vi "运维调试_五参数.vi"() -> ()   [LabVIEW 2016, in "斯坦道多参数.lvlib"]
uses:
  <vilib>/Utility/miscctls.llb/LVPointTypeDef.ctl
  <vilib>/Utility/config.llb/NI_LVConfig.lvlib
panel:
  in  "周期设置":bool
  in  "序号":string
  out "字符串":string
  out "运行状态":u16(ring) items=["空闲", "水样测试", "标样核查"]
  in  "叶绿素a校准":bool
  in  "停止":bool
  in  "标样核查":bool
  in  "水样测试":bool
  in  "open MB":bool
  in  "设置":bool
  in  "水温校准":bool
  in  "浊度校准":bool
  in  "溶解氧校准":bool
  in  "电导率校准":bool
  in  "pH校准":bool
  in  "探头校正返回":bool
  in  "探头校正":bool
  out "检测值":T1
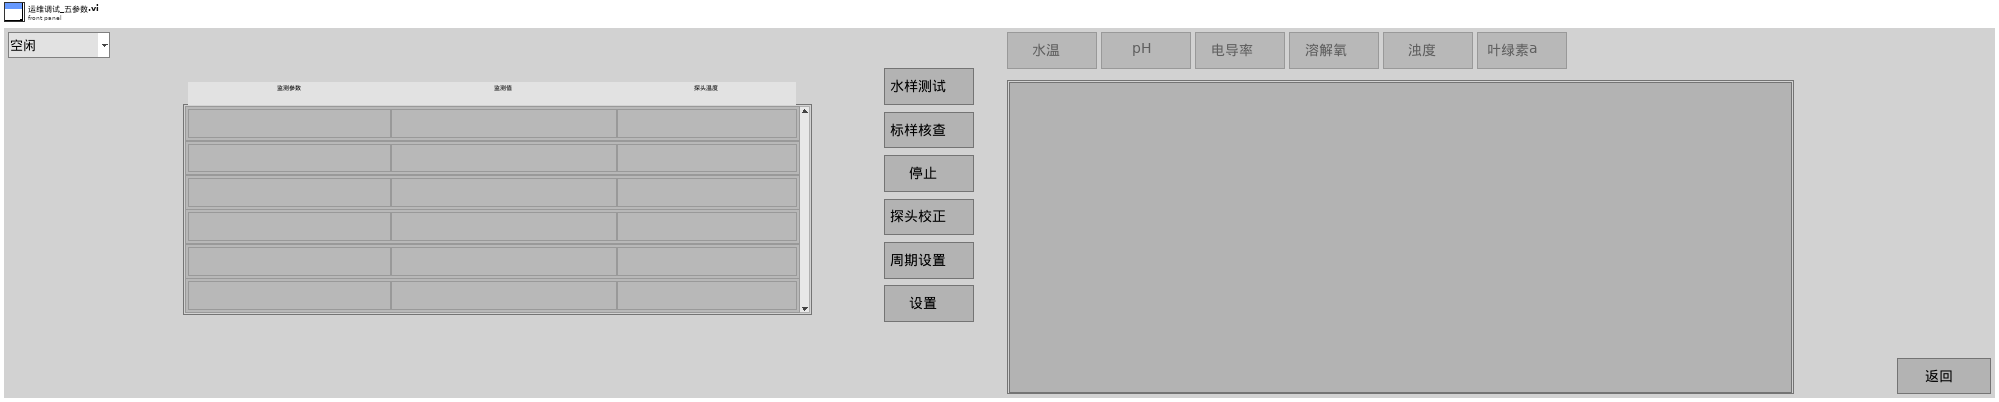
[diagram p1: front panel]
types:
  T1 = typedef "斯坦道多参数.lvlib/检测值.ctl" = cluster{"监测参数1":string, "浓度1":string, "探头温度1":string}[]
  T2 = typedef "LVPointTypeDef.ctl" = cluster{"Horizontal":i16, "Vertical":i16}
  T3 = cluster{"电极状态标志":u16, "电极型号标志":u16, "溶解氧测量值":sgl, "温度测量值":sgl, "溶解氧饱和度值":sgl, "盐度补偿值":sgl, "大气压补偿值":sgl, "溶解氧偏移修正值":sgl, "温度偏移修正值":sgl, "手动温度补偿值":sgl, "溶解氧电极零点":sgl, "溶解氧电极斜率":sgl, "第1点标准值记录":sgl, "第1点信号值记录":sgl, "第1点温度值记录":sgl, "第2点标准值记录":sgl, "第2点信号值记录":sgl, "第2点温度值记录":sgl, "命令滤波设定":u16, "温度模式":enum16{"ATC", "MTC"}, "生产批次":u16, "电极序号":u16, "串口地址":u16, "串口波特率":enum16{"9600", "19200", "115200"}, "串口校验位":enum16{"NONE", "ODD", "EVEN"}, "串口停止位":enum16{"1bit", "2bit"}, "第一点标准值":sgl, "第二点标准值":sgl}
  T4 = cluster{"电极状态标志":u16, "电极型号标志":u16, "酸碱度测量值":sgl, "温度测量值":sgl, "酸碱度信号值":sgl, "温度信号值":sgl, "酸碱度偏移修正值":sgl, "温度偏移修正值":sgl, "手动温度补偿值":sgl, "酸碱度电极零点":sgl, "酸碱度电极斜率":sgl, "第1点标准值记录":sgl, "第1点信号值记录":sgl, "第1点温度值记录":sgl, "第2点标准值记录":sgl, "第2点信号值记录":sgl, "第2点温度值记录":sgl, "命令滤波设定":u16, "温度模式":enum16{"ATC", "MTC"}, "生产批次":u16, "电极序号":u16, "串口地址":u16, "串口波特率":enum16{"9600", "19200", "115200"}, "串口校验位":enum16{"NONE", "ODD", "EVEN"}, "串口停止位":enum16{"1bit", "2bit"}, "第一点标准值":sgl, "第二点标准值":sgl}
  T5 = cluster{"电极状态标志":u16, "电极型号标志":u16, "浊度测量值":sgl, "温度测量值":sgl, "浊度信号值":sgl, "浊度偏移修正值":sgl, "温度偏移修正值":sgl, "手动温度补偿值":sgl, "浊度电极零点":sgl, "浊度电极斜率":sgl, "第1点标准值记录":sgl, "第1点信号值记录":sgl, "第1点温度值记录":sgl, "第2点标准值记录":sgl, "第2点信号值记录":sgl, "第2点温度值记录":sgl, "命令滤波设定":u16, "温度模式":enum16{"ATC", "MTC"}, "生产批次":u16, "电极序号":u16, "串口地址":u16, "串口波特率":enum16{"9600", "19200", "115200"}, "串口校验位":enum16{"NONE", "ODD", "EVEN"}, "串口停止位":enum16{"1bit", "2bit"}, "第一点标准值":sgl, "第二点标准值":sgl}
  T6 = cluster{"电极状态标志":u16, "电极型号标志":u16, "电导率测量值":sgl, "温度测量值":sgl, "电导率信号值":sgl, "温度信号值":sgl, "温度补偿系数":sgl, "电导率偏移修正值":sgl, "温度偏移修正值":sgl, "手动温度补偿值":sgl, "电导率电极零点":sgl, "电导率电极斜率":sgl, "命令滤波设定":u16, "温度模式":enum16{"ATC", "MTC"}, "生产批次":u16, "电极序号":u16, "串口地址":u16, "串口波特率":enum16{"9600", "19200", "115200"}, "串口校验位":enum16{"NONE", "ODD", "EVEN"}, "串口停止位":enum16{"1bit", "2bit"}, "第一点标准值":sgl, "第二点标准值":sgl}
  T7 = cluster{"监测参数1":string, "浓度1":string, "探头温度1":string}[]
  T8 = enum8{"Enabled", "Disabled", "Disabled and Grayed Out"}
  T9 = cluster{"CH":u16, "监测值":dbl, "监测信号值":dbl, "温度偏移修正值":sgl}
  T10 = typedef "NI_LVConfig.lvlib/Config Data RefNum.ctl" = refnum<k1>
  T11 = enum32{"Bad", "Idle", "Run top level", "Running"}
  T12 = enum32{"Invalid", "Standard", "Closed", "Hidden", "Minimized", "Maximized"}
  T13 = cluster{"数据保存间隔":dbl, "水温标样值":dbl, "pH标样值":dbl, "溶解氧标样值":dbl, "电导率标样值":dbl, "浊度标样值":dbl}
  T14 = cluster{"Temp":bool, "pH":bool, "DO":bool, "Cond":bool, "Turb":bool, "叶绿素a启用":bool, "蓝绿藻":bool}
  T15 = cluster{"baud rate (bps)":u32, "stop bits":u16, "parity":u16, "flow control":u16, "timeout":u32, "retries":i32}
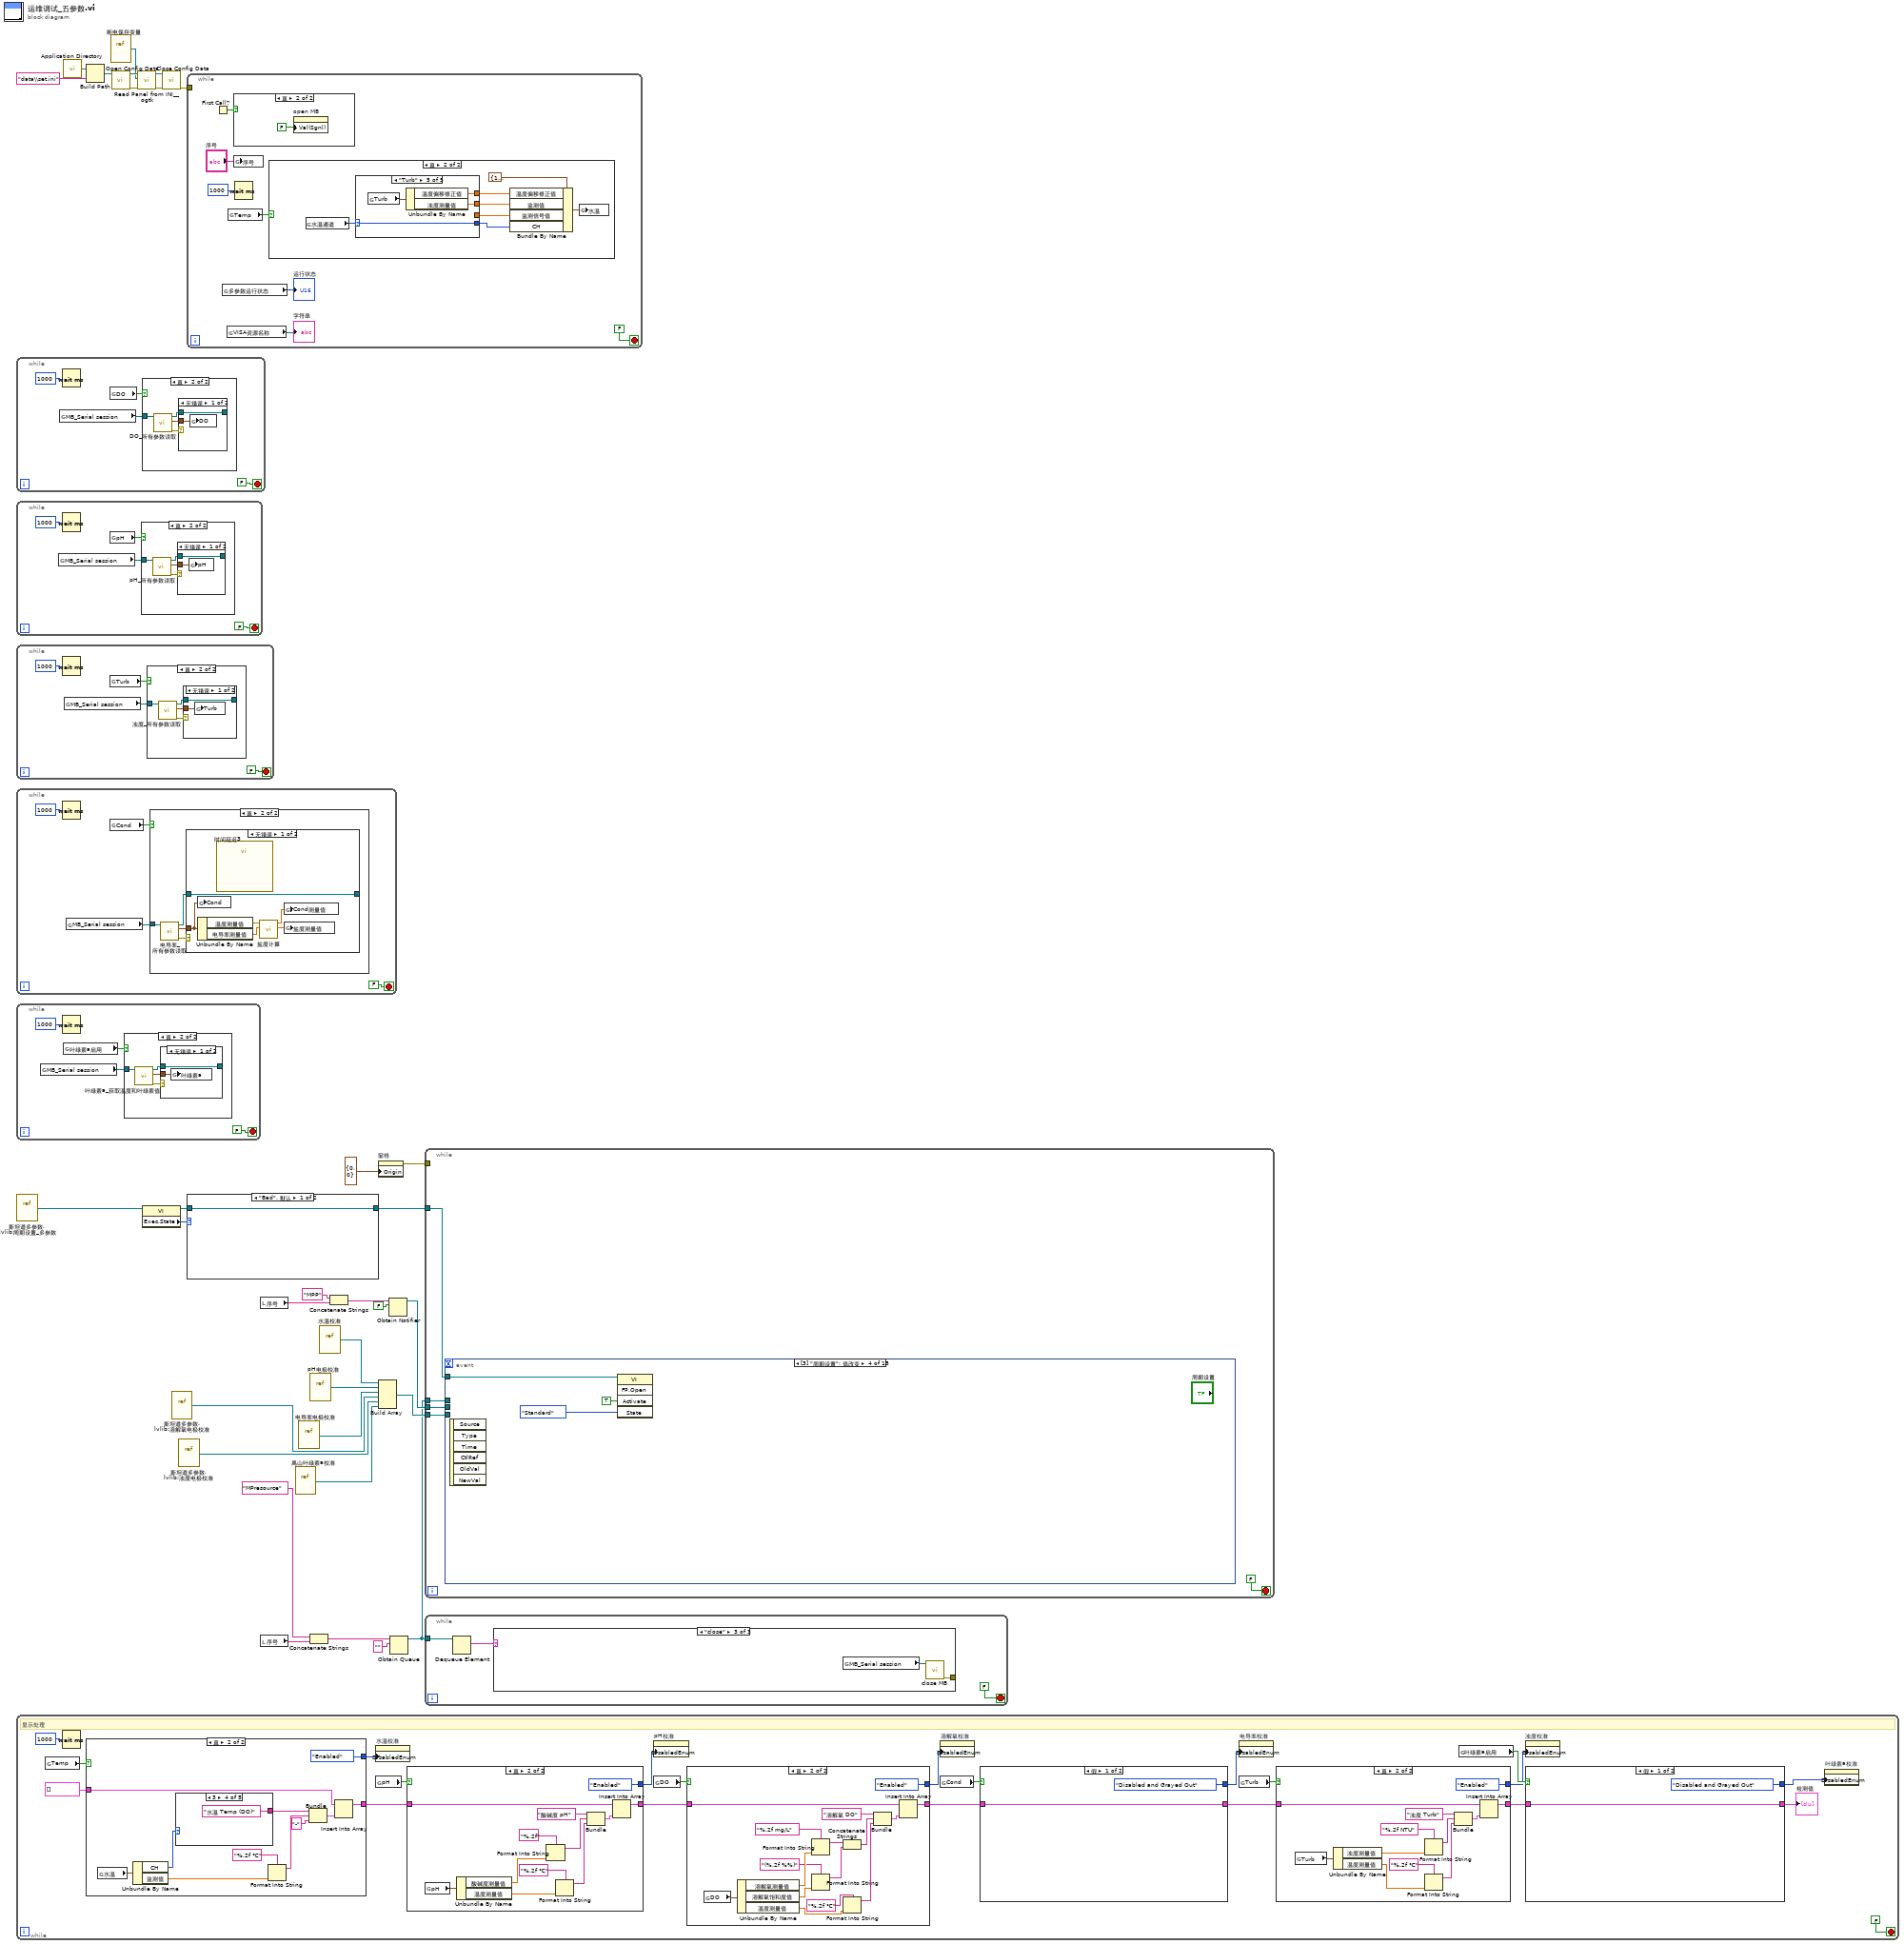
[diagram p0: block diagram]
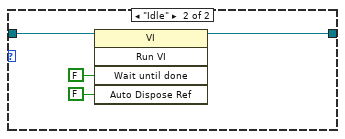
[diagram p2: hidden frame]
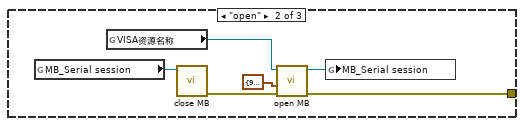
[diagram p4: hidden frame]
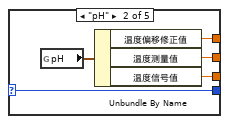
[diagram p17: hidden frame]
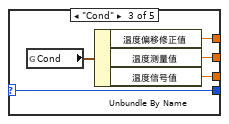
[diagram p18: hidden frame]
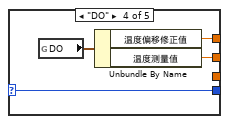
[diagram p19: hidden frame]
diagram:
  n1 = while {
    stop <- FALSE stop-if-true
    n2 = global read "多参数全局变量.vi" "MB_Serial session"() -> (w33:refnum<class "MB_Master_Serial.lvclass">)
    n3 = Wait (ms)(milliseconds to wait=u32 1000 ("等待时间（毫秒）")) -> ()  [unwired: 1 out]
    n4 = global read "断电保存变量.vi" "DO"() -> (w34:bool)
    n5 = case shown="真" w34 {
      tunnel: w33 -> [_ w37]
      frame False {
      }
      frame True {
        n6 = call "DO_所有参数读取.vi"("MB_Serial session in"=w37) -> ("error out"=w39:errorcluster, "输出值"=w40:T3, "MB_Serial session out"=w38:refnum<class "MB_Master_Serial.lvclass">)  [unwired: 8 in]
        n7 = case shown="无错误" w39 {
          tunnel: w40 -> [w41 _]
          tunnel: w38 -> [w42 w43]
          tunnel: [w42 w43] -> _
          frame No Error {
            n8 = global write "国弘过程全局变量.vi" "DO"(w41) -> ()
          }
          frame Error {
          }
        }
      }
    }
  }
  n9 = while {
    stop <- FALSE stop-if-true
    n10 = global read "多参数全局变量.vi" "MB_Serial session"() -> (w44:refnum<class "MB_Master_Serial.lvclass">)
    n11 = Wait (ms)(milliseconds to wait=u32 1000 ("等待时间（毫秒）")) -> ()  [unwired: 1 out]
    n12 = global read "断电保存变量.vi" "pH"() -> (w46:bool)
    n13 = case shown="真" w46 {
      tunnel: w44 -> [_ w48]
      frame False {
      }
      frame True {
        n14 = call "pH_所有参数读取.vi"("MB_Serial session in"=w48) -> ("error out"=w50:errorcluster, "输出值"=w51:T4, "MB_Serial session out"=w49:refnum<class "MB_Master_Serial.lvclass">)  [unwired: 8 in]
        n15 = case shown="无错误" w50 {
          tunnel: w51 -> [w53 _]
          tunnel: w49 -> [w52 w54]
          tunnel: [w52 w54] -> _
          frame No Error {
            n16 = global write "国弘过程全局变量.vi" "pH"(w53) -> ()
          }
          frame Error {
          }
        }
      }
    }
  }
  n17 = while {
    stop <- FALSE stop-if-true
    n18 = Wait (ms)(milliseconds to wait=u32 1000 ("等待时间（毫秒）")) -> ()  [unwired: 1 out]
    n19 = global read "多参数全局变量.vi" "MB_Serial session"() -> (w55:refnum<class "MB_Master_Serial.lvclass">)
    n20 = global read "断电保存变量.vi" "Turb"() -> (w57:bool)
    n21 = case shown="真" w57 {
      tunnel: w55 -> [_ w59]
      frame False {
      }
      frame True {
        n22 = call "浊度_所有参数读取.vi"("MB_Serial session in"=w59) -> ("error out"=w61:errorcluster, "输出值"=w62:T5, "MB_Serial session out"=w60:refnum<class "MB_Master_Serial.lvclass">)  [unwired: 8 in]
        n23 = case shown="无错误" w61 {
          tunnel: w62 -> [w63 _]
          tunnel: w60 -> [w64 w65]
          tunnel: [w64 w65] -> _
          frame No Error {
            n24 = global write "国弘过程全局变量.vi" "Turb"(w63) -> ()
          }
          frame Error {
          }
        }
      }
    }
  }
  n25 = while {
    stop <- FALSE stop-if-true
    n26 = Wait (ms)(milliseconds to wait=u32 1000 ("等待时间（毫秒）")) -> ()  [unwired: 1 out]
    n27 = global read "多参数全局变量.vi" "MB_Serial session"() -> (w66:refnum<class "MB_Master_Serial.lvclass">)
    n28 = global read "断电保存变量.vi" "Cond"() -> (w68:bool)
    n29 = case shown="真" w68 {
      tunnel: w66 -> [_ w70]
      frame False {
      }
      frame True {
        n30 = call "电导率_所有参数读取.vi"("MB_Serial session in"=w70) -> ("error out"=w72:errorcluster, "输出值"=w73:T6, "MB_Serial session out"=w71:refnum<class "MB_Master_Serial.lvclass">)  [unwired: 8 in]
        n31 = case shown="无错误" w72 {
          tunnel: w73 -> [w78 _]
          tunnel: [w79 w80] -> _
          tunnel: w71 -> [w79 w80]
          frame No Error {
            n32 = global write "国弘过程全局变量.vi" "Cond"(w78) -> ()
            n33 = Unbundle By Name(w78) -> ("温度测量值"=w76:sgl, "电导率测量值"=w77:sgl)
            n34 = call "时间延迟3"() -> ()  [unwired: 11 in, 1 out]
            n35 = call "盐度计算.vi"("spCond"=w77, "Temp"=w76) -> ("saltresult"=w74:dbl, "cond"=w75:dbl)  [unwired: 8 in]
            n36 = global write "国弘过程全局变量.vi" "Cond测量值"(w75) -> ()
            n37 = global write "国弘过程全局变量.vi" "盐度测量值"(w74) -> ()
          }
          frame Error {
          }
        }
      }
    }
  }
  n38 = while {
    stop <- FALSE stop-if-true
    n39 = global read "多参数全局变量.vi" "MB_Serial session"() -> (w81:refnum<class "MB_Master_Serial.lvclass">)
    n40 = Wait (ms)(milliseconds to wait=u32 1000 ("等待时间（毫秒）")) -> ()  [unwired: 1 out]
    n41 = global read "断电保存变量.vi" "叶绿素a启用"() -> (w83:bool)
    n42 = case shown="真" w83 {
      tunnel: w81 -> [_ w85]
      frame False {
      }
      frame True {
        n43 = call "叶绿素a_获取温度和叶绿素值.vi"("MB_Serial session in"=w85) -> ("error out"=w87:errorcluster, "输出值"=w88:cluster{"温度测量值":sgl, "叶绿素测量值":sgl, "错误标志":u16}, "MB_Serial session out"=w86:refnum<class "MB_Master_Serial.lvclass">)  [unwired: 8 in]
        n44 = case shown="无错误" w87 {
          tunnel: w88 -> [w89 _]
          tunnel: w86 -> [w90 w91]
          tunnel: [w90 w91] -> _
          frame No Error {
            n45 = global write "禹山过程全局变量.vi" "叶绿素a"(w89) -> ()
          }
          frame Error {
          }
        }
      }
    }
  }
  n46 = vi-ref "斯坦道多参数.lvlib:周期设置_多参数.vi"() -> (w4:refnum<vi>)
  n47 = while {
    stop <- FALSE stop-if-true
    # "显示处理"
    n48 = global read "断电保存变量.vi" "Temp"() -> (w110:bool)
    n49 = Wait (ms)(milliseconds to wait=u32 1000 ("等待时间（毫秒）")) -> ()  [unwired: 1 out]
    n50 = case shown="真" w110 {
      tunnel: [w188 w190] -> w107
      tunnel: T7 [] ("数组") -> [w188 w191]
      tunnel: [T8."Disabled and Grayed Out" ("禁用") T8."Enabled" ("禁用")] -> w92
      frame False {
      }
      frame True {
        n51 = global read "国弘过程全局变量.vi" "水温"() -> (w199:T9)
        n52 = Unbundle By Name(w199) -> ("CH"=w196:u16, "监测值"=w197:dbl)
        n53 = case shown="3" w196 {
          tunnel: ["水温 Temp" ("监测参数1") "水温 Temp (pH)" ("监测参数1") "水温 Temp (Cond)" ("监测参数1") "水温 Temp (DO)" ("监测参数1") "水温 Temp (Turb)" ("监测参数1")] -> w195
          frame 0, Default {
          }
          frame 1 {
          }
          frame 2 {
          }
          frame 3 {
          }
          frame 4 {
          }
        }
        n54 = Format Into String(format string="%.2f ℃" ("格式字符串"), w197) -> (resulting string=w194:string)  [unwired: 2 in, 1 out]
        n55 = Bundle("监测参数1"=w195, w194, "探头温度1"="-") -> (w192:cluster{"监测参数1":string, string, "探头温度1":string})  [unwired: 1 in]
        n56 = Insert Into Array(array=w191, new element=w192) -> (w190:T7)  [unwired: 1 in]
      }
    }
    n57 = property on="水温校准" class="Bool"("DisabledEnum"=w92) -> ()  [unwired: 2 in, 2 out]
    n58 = global read "断电保存变量.vi" "pH"() -> (w108:bool)
    n59 = case shown="真" w108 {
      tunnel: [w174 w176] -> w105
      tunnel: w107 -> [w174 w178]
      tunnel: [T8."Disabled and Grayed Out" ("禁用") T8."Enabled" ("禁用")] -> w97
      frame False {
      }
      frame True {
        n60 = global read "国弘过程全局变量.vi" "pH"() -> (w186:T4)
        n61 = Unbundle By Name(w186) -> ("酸碱度测量值"=w185:sgl, "温度测量值"=w183:sgl)
        n62 = Format Into String(format string="%.2f" ("格式字符串"), w185) -> (resulting string=w179:string)  [unwired: 2 in, 1 out]
        n63 = Format Into String(format string="%.2f ℃" ("格式字符串"), w183) -> (resulting string=w181:string)  [unwired: 2 in, 1 out]
        n64 = Bundle("监测参数2"="酸碱度 pH", w179, w181) -> (w177:cluster{"监测参数2":string, string, string})  [unwired: 1 in]
        n65 = Insert Into Array(array=w178, new element=w177) -> (w176:T7)  [unwired: 1 in]
      }
    }
    n66 = property on="pH校准" class="Bool"("DisabledEnum"=w97) -> ()  [unwired: 2 in, 2 out]
    n67 = global read "断电保存变量.vi" "DO"() -> (w106:bool)
    n68 = case shown="真" w106 {
      tunnel: [w156 w159] -> w102
      tunnel: w105 -> [w156 w160]
      tunnel: [T8."Disabled and Grayed Out" ("禁用") T8."Enabled" ("禁用")] -> w96
      frame False {
      }
      frame True {
        n69 = global read "国弘过程全局变量.vi" "DO"() -> (w157:T3)
        n70 = Unbundle By Name(w157) -> ("溶解氧测量值"=w169:sgl, "溶解氧饱和度值"=w167:sgl, "温度测量值"=w171:sgl)
        n71 = Format Into String(format string="%.2f mg/L" ("格式字符串"), w169) -> (resulting string=w166:string)  [unwired: 2 in, 1 out]
        n72 = Format Into String(format string="(%.2f %%)" ("格式字符串"), w167) -> (resulting string=w165:string)  [unwired: 2 in, 1 out]
        n73 = Concatenate Strings(w166, w165) -> (w164:string)
        n74 = Format Into String(format string="%.2f ℃" ("格式字符串"), w171) -> (resulting string=w162:string)  [unwired: 2 in, 1 out]
        n75 = Bundle("监测参数2"="溶解氧 DO", w164, w162) -> (w161:cluster{"监测参数2":string, string, string})  [unwired: 1 in]
        n76 = Insert Into Array(array=w160, new element=w161) -> (w159:T7)  [unwired: 1 in]
      }
    }
    n77 = property on="溶解氧校准" class="Bool"("DisabledEnum"=w96) -> ()  [unwired: 2 in, 2 out]
    n78 = global read "断电保存变量.vi" "Cond"() -> (w104:bool)
    n79 = case shown="假" w104 {
      tunnel: w102 -> [w142 w146]
      tunnel: [w142 w144] -> w101
      tunnel: [T8."Disabled and Grayed Out" ("禁用") T8."Enabled" ("禁用")] -> w95
      frame False {
      }
      frame True {
        n80 = global read "国弘过程全局变量.vi" "Cond"() -> (w154:T6)
        n81 = Unbundle By Name(w154) -> ("电导率测量值"=w153:sgl, "温度测量值"=w151:sgl)
        n82 = Format Into String(format string="%.2f uS/cm" ("格式字符串"), w153) -> (resulting string=w147:string)  [unwired: 2 in, 1 out]
        n83 = Format Into String(format string="%.2f ℃" ("格式字符串"), w151) -> (resulting string=w148:string)  [unwired: 2 in, 1 out]
        n84 = Bundle("监测参数2"="电导率 Cond", w147, w148) -> (w145:cluster{"监测参数2":string, string, string})  [unwired: 1 in]
        n85 = Insert Into Array(array=w146, new element=w145) -> (w144:T7)  [unwired: 1 in]
      }
    }
    n86 = property on="电导率校准" class="Bool"("DisabledEnum"=w95) -> ()  [unwired: 2 in, 2 out]
    n87 = global read "断电保存变量.vi" "Turb"() -> (w103:bool)
    n88 = case shown="真" w103 {
      tunnel: w101 -> [w128 w133]
      tunnel: [w128 w131] -> w100
      tunnel: [T8."Disabled and Grayed Out" ("禁用") T8."Enabled" ("禁用")] -> w94
      frame False {
      }
      frame True {
        n89 = global read "国弘过程全局变量.vi" "Turb"() -> (w129:T5)
        n90 = Unbundle By Name(w129) -> ("浊度测量值"=w137:sgl, "温度测量值"=w139:sgl)
        n91 = Format Into String(format string="%.2f NTU" ("格式字符串"), w137) -> (resulting string=w135:string)  [unwired: 2 in, 1 out]
        n92 = Format Into String(format string="%.2f ℃" ("格式字符串"), w139) -> (resulting string=w136:string)  [unwired: 2 in, 1 out]
        n93 = Bundle("监测参数2"="浊度 Turb", w135, w136) -> (w132:cluster{"监测参数2":string, string, string})  [unwired: 1 in]
        n94 = Insert Into Array(array=w133, new element=w132) -> (w131:T7)  [unwired: 1 in]
      }
    }
    n95 = global read "断电保存变量.vi" "叶绿素a启用"() -> (w98:bool)
    n96 = property on="浊度校准" class="Bool"("DisabledEnum"=w94) -> ()  [unwired: 2 in, 2 out]
    n97 = case shown="假" w98 {
      tunnel: w100 -> [w114 w121]
      tunnel: [w114 w119] -> w99
      tunnel: [T8."Disabled and Grayed Out" ("禁用") T8."Enabled" ("禁用")] -> w93
      frame False {
      }
      frame True {
        n98 = global read "禹山过程全局变量.vi" "叶绿素a"() -> (w118:cluster{"温度测量值":sgl, "叶绿素测量值":sgl, "错误标志":u16})
        n99 = Unbundle By Name(w118) -> ("叶绿素测量值"=w117:sgl, "温度测量值"=w116:sgl)
        n100 = Format Into String(format string="%.2f ug/L" ("格式字符串"), w117) -> (resulting string=w123:string)  [unwired: 2 in, 1 out]
        n101 = Format Into String(format string="%.2f ℃" ("格式字符串"), w116) -> (resulting string=w124:string)  [unwired: 2 in, 1 out]
        n102 = Bundle("监测参数2"="叶绿素a Chla", w123, w124) -> (w120:cluster{"监测参数2":string, string, string})  [unwired: 1 in]
        n103 = Insert Into Array(array=w121, new element=w120) -> (w119:T7)  [unwired: 1 in]
      }
    }
    "检测值" <- w99
    n104 = property on="叶绿素a校准" class="Bool"("DisabledEnum"=w93) -> ()  [unwired: 2 in, 2 out]
  }
  n105 = call <vilib>:"Application Directory.vi"() -> ("Application Directory"=w20:path)
  n106 = Build Path(base path=w20, name or relative path="data\\set.ini" ("名称或相对路径")) -> (appended path=w19:path)
  n107 = vi-ref "断电保存变量.vi"() -> (w17:refnum<vi>)
  n108 = call <vilib>:"Open Config Data.vi"("configuration file path"=w19) -> ("error out"=w23:errorcluster, "refnum"=w24:T10)  [unwired: 8 in, 1 out]
  n109 = call <userlib>:"Read Panel from INI__ogtk.vi"("error in (no error)"=w23, "VI ref"=w17, "refnum"=w24) -> ("error out"=w21:errorcluster, "refnum out"=w22:T10)  [unwired: 7 in]
  n110 = property class="VI"(reference=w4) -> (reference out=w2:refnum<vi>, "Exec.State"=w3:T11)  [unwired: 1 in, 1 out]
  n111 = call <vilib>:"Close Config Data.vi"("error in (no error)"=w21, "refnum"=w22) -> ("error out"=w16:errorcluster)  [unwired: 8 in, 1 out]
  n112 = vi-ref "斯坦道多参数.lvlib:溶解氧电极校准.vi"() -> (w26:refnum<vi>)
  n113 = vi-ref "斯坦道多参数.lvlib:浊度电极校准.vi"() -> (w25:refnum<vi>)
  n114 = while {
    tunnel: w16 -> [_]
    stop <- FALSE stop-if-true
    n115 = First Call?() -> (First Call?: T/F=w209:bool)
    n116 = global read "多参数全局变量.vi" "多参数运行状态"() -> (→"运行状态":u16)
    n117 = global read "断电保存变量.vi" "VISA资源名称"() -> (→"字符串":refnum<visa-resource-name>)
    n118 = global read "断电保存变量.vi" "Temp"() -> (w208:bool)
    n119 = case shown="真" w209 {
      frame False {
      }
      frame True {
        n120 = property on="open MB" class="Bool (严格)"("Val(Sgnl)"=FALSE ("值(信号)")) -> ()  [unwired: 2 in, 2 out]
      }
    }
    n121 = global write "多参数全局变量.vi" "序号"("序号") -> ()
    n122 = Wait (ms)(milliseconds to wait=u32 1000 ("等待时间（毫秒）")) -> ()  [unwired: 1 out]
    n123 = case shown="真" w208 {
      frame False {
      }
      frame True {
        n124 = global read "断电保存变量.vi" "水温通道"() -> (w218:enum16{"NULL", "pH", "Cond", "DO", "Turb"})
        n125 = case shown="\"Turb\"" w218 {
          selector: w218 -> [w219 w224 w229 w233 w237]
          tunnel: [w219 w224 w229 w233 w237] -> w217
          tunnel: [_ w222 w227 w230 w235] -> w216
          tunnel: [_ w221 w226 _ _] -> w215
          tunnel: [_ w220 w225 w231 w234] -> w212
          frame "NULL", Default {
          }
          frame "pH" {
            n126 = global read "国弘过程全局变量.vi" "pH"() -> (w223:T4)
            n127 = Unbundle By Name(w223) -> ("温度偏移修正值"=w220:sgl, "温度测量值"=w222:sgl, "温度信号值"=w221:sgl)
          }
          frame "Cond" {
            n128 = global read "国弘过程全局变量.vi" "Cond"() -> (w228:T6)
            n129 = Unbundle By Name(w228) -> ("温度偏移修正值"=w225:sgl, "温度测量值"=w227:sgl, "温度信号值"=w226:sgl)
          }
          frame "DO" {
            n130 = global read "国弘过程全局变量.vi" "DO"() -> (w232:T3)
            n131 = Unbundle By Name(w232) -> ("温度偏移修正值"=w231:sgl, "温度测量值"=w230:sgl)
          }
          frame "Turb" {
            n132 = global read "国弘过程全局变量.vi" "Turb"() -> (w236:T5)
            n133 = Unbundle By Name(w236) -> ("温度偏移修正值"=w234:sgl, "浊度测量值"=w235:sgl)
          }
        }
        n134 = Bundle By Name(cluster=T9 {"CH"=1, "监测值"=0.0, "监测信号值"=0.0, "温度偏移修正值"=0.0} ("水温"), "温度偏移修正值"=w212, "监测值"=w216, "监测信号值"=w215, "CH"=w217) -> (w214:T9)
        n135 = global write "国弘过程全局变量.vi" "水温"(w214) -> ()
      }
    }
  }
  n136 = case shown="\"Bad\", 默认" w3 {
    tunnel: w2 -> [w239 w243]
    tunnel: [w239 w240] -> w1
    frame "Bad", Default {
    }
    frame "Idle" {
      n137 = invoke class="VI" method="Run VI"(reference=w243, "Wait until done"=FALSE ("结束前等待"), "Auto Dispose Ref"=FALSE ("自动销毁引用")) -> (reference out=w240:refnum<vi>)  [unwired: 2 in, 4 out]
    }
  }
  n138 = local read "序号"() -> (w6:string)
  n139 = local read "序号"() -> (w5:string)
  n140 = vi-ref "禹山叶绿素a校准.vi"() -> (w15:refnum<vi>)
  n141 = vi-ref "电导率电极校准.vi"() -> (w27:refnum<vi>)
  n142 = Concatenate Strings("MPresource" ("名称（未命名）"), w5) -> (w7:string)
  n143 = vi-ref "pH电极校准.vi"() -> (w28:refnum<vi>)
  n144 = vi-ref "水温校准.vi"() -> (w29:refnum<vi>)
  n145 = Concatenate Strings("MPP" ("名称（未命名）"), w6) -> (w8:string)
  n146 = property on="窗格" class="Pane"("Origin"=T2 {"Horizontal"=0, "Vertical"=0} ("原点")) -> (error out=w32:errorcluster)  [unwired: 2 in, 1 out]
  n147 = Build Array(w29, w28, w27, w26, w25, w15) -> (w30:refnum<vi>[])
  n148 = Obtain Notifier(name (unnamed)=w8, notification data type=FALSE) -> (notifier out=w12:refnum<notifier>)  [unwired: 2 in, 2 out]
  n149 = Obtain Queue(name (unnamed)=w7, element data type="" ("名称（未命名）")) -> (queue out=w9:refnum<queue>)  [unwired: 3 in, 2 out]
  n150 = while {
    tunnel: w32 -> [_]
    tunnel: w30 -> [w247]
    tunnel: w12 -> [w246]
    tunnel: w9 -> [w245]
    tunnel: w1 -> [w244]
    stop <- FALSE stop-if-true
    n151 = event shown="[3] \"周期设置\": 值改变" {
      selector: _ -> [_ _ _ _ _ _ _ _ _ _ _ _ _ _ _]
      dyn-events: _ -> [_ _ _ _ _ _ _ _ _ _ _ _ _ _ _]
      timeout: _ -> [_ _ _ _ _ _ _ _ _ _ _ _ _ _ _]
      tunnel: w247 -> [_ _ _ _ _ _ _ w310 w323 w336 w348 w360 w372 w384 w396]
      tunnel: w246 -> [_ _ _ _ w283 _ _ _ _ _ _ _ _ _ _]
      tunnel: w245 -> [_ _ _ _ _ w286 _ _ _ _ _ _ _ _ _]
      tunnel: w244 -> [_ _ _ w281 _ _ _ _ _ _ _ _ _ _ _]
      event Timeout {
        n152 = event-data() -> ()  [unwired: 1 in, 3 out]
      }
      event "水样测试": Value Change {
        n153 = event-data() -> ()  [unwired: 1 in, 6 out]
        n154 = call "水样测试配置.vi"() -> ("确认输出"=w250:bool, "水样测定时间输出"=w249:dbl)  [unwired: 10 in]
        n155 = case shown="真" w250 {
          tunnel: w249 -> [_ w253]
          frame False {
          }
          frame True {
            n156 = vi-ref "水样测试.vi"() -> (w254:refnum<vi>)
            n157 = property class="VI"(reference=w254) -> ("Name"=w258:string, "Exec.State"=w256:T11)  [unwired: 1 in, 2 out]
            n158 = Open VI Reference(type specifier VI Refnum (for type only)=refnum<vi> refnum, vi path=w258, options=128 ("选项")) -> (vi reference=w259:refnum<vi>)  [unwired: 3 in, 1 out]
            n159 = case shown="\"Idle\"" w256 {
              tunnel: [w260 w264] -> w255
              tunnel: w259 -> [w260 w263]
              tunnel: w253 -> [_ w262]
              tunnel: "hd" ("数据标记表") -> [_ w261]
              frame "Bad", Default {
              }
              frame "Idle" {
                n160 = call-by-ref "开始异步调用"(reference=w263, "数据标记表"=w261, "水样测试时间"=w262) -> (reference out=w264:refnum<vi>)  [unwired: 11 in, 1 out]
              }
            }
            n161 = Close Reference(reference=w255) -> ()  [unwired: 1 in, 1 out]
          }
        }
      }
      event "标样核查": Value Change {
        n162 = event-data() -> ()  [unwired: 1 in, 6 out]
        n163 = call "标样核查配置.vi"() -> ("确认输出"=w266:bool, "标样核查配置"=w265:T13)  [unwired: 10 in]
        n164 = case shown="真" w266 {
          tunnel: w265 -> [_ w267]
          frame False {
          }
          frame True {
            n165 = vi-ref "标样核查.vi"() -> (w268:refnum<vi>)
            n166 = property class="VI"(reference=w268) -> ("Name"=w273:string, "Exec.State"=w270:T11)  [unwired: 1 in, 2 out]
            n167 = Open VI Reference(type specifier VI Refnum (for type only)=refnum<vi> refnum, vi path=w273, options=128 ("选项")) -> (vi reference=w274:refnum<vi>)  [unwired: 3 in, 1 out]
            n168 = case shown="\"Idle\"" w270 {
              tunnel: [w275 w278] -> w269
              tunnel: w274 -> [w275 w277]
              tunnel: w267 -> [_ w276]
              frame "Bad", Default {
              }
              frame "Idle" {
                n169 = call-by-ref "开始异步调用"(reference=w277, "标样核查配置"=w276) -> (reference out=w278:refnum<vi>)  [unwired: 12 in, 1 out]
              }
            }
            n170 = Close Reference(reference=w269) -> ()  [unwired: 1 in, 1 out]
          }
        }
      }
      event "周期设置": Value Change {
        n171 = event-data() -> ()  [unwired: 1 in, 6 out]
        n172 = invoke class="VI" method="FP.Open"(reference=w281, "Activate"=TRUE ("激活？"), "State"=T12."Standard" ("状态")) -> ()  [unwired: 2 in, 5 out]
      }
      event "停止": Value Change {
        n173 = event-data() -> ()  [unwired: 1 in, 6 out]
        n174 = Send Notification(notification=TRUE ("通知"), notifier=w283) -> ()  [unwired: 1 in, 2 out]
      }
      event "open MB": Value Change {
        n175 = event-data() -> ()  [unwired: 1 in, 6 out]
        n176 = Flush Queue(queue=w286) -> (queue out=w285:refnum<queue>)  [unwired: 1 in, 2 out]
        n177 = Enqueue Element(queue=w285, element="open" ("元素")) -> ()  [unwired: 2 in, 3 out]
      }
      event "设置": Value Change {
        n178 = event-data() -> ()  [unwired: 1 in, 6 out]
        n179 = flat-sequence {
          frame #0 {
            n180 = call "配置.vi"() -> ("启用参数"=w294:T14, "串口输出"=w295:refnum<visa-resource-name>)  [unwired: 10 in]
            n181 = global write "断电保存变量.vi" "VISA资源名称"(w295) -> ()
            n182 = Unbundle By Name(w294) -> ("Temp"=w289:bool, "pH"=w290:bool, "DO"=w291:bool, "Cond"=w292:bool, "Turb"=w293:bool, "叶绿素a启用"=w288:bool, "蓝绿藻"=w287:bool)
            n183 = global write "断电保存变量.vi" "pH"(w290) -> ()
            n184 = global write "断电保存变量.vi" "DO"(w291) -> ()
            n185 = global write "断电保存变量.vi" "Cond"(w292) -> ()
            n186 = global write "断电保存变量.vi" "Turb"(w293) -> ()
            n187 = global write "断电保存变量.vi" "Temp"(w289) -> ()
            n188 = global write "断电保存变量.vi" "叶绿素a启用"(w288) -> ()
            n189 = global write "断电保存变量.vi" "蓝绿藻"(w287) -> ()
          }
          frame #1 {
            n190 = call <vilib>:"Application Directory.vi"() -> ("Application Directory"=w305:path)
            n191 = Build Path(base path=w305, name or relative path="data\\set.ini" ("名称或相对路径")) -> (appended path=w304:path)
            n192 = call <vilib>:"Open Config Data.vi"("configuration file path"=w304) -> ("error out"=w308:errorcluster, "refnum"=w309:T10)  [unwired: 8 in, 1 out]
            n193 = vi-ref "断电保存变量.vi"() -> (w302:refnum<vi>)
            n194 = call <userlib>:"Write Panel to INI__ogtk.vi"("error in (no error)"=w308, "VI ref"=w302, "refnum"=w309) -> ("error out"=w306:errorcluster, "refnum out"=w307:T10)  [unwired: 7 in]
            n195 = call <vilib>:"Close Config Data.vi"("error in (no error)"=w306, "refnum"=w307) -> ("error out"=w298:errorcluster, "file path"=w299:path)  [unwired: 8 in]
            n196 = Open/Create/Replace File(file path (use dialog)=w299, error in=w298) -> (refnum out=w300:refnum<file>, error out=w301:errorcluster)  [unwired: 4 in, 1 out]
            n197 = Flush File(refnum=w300, error in=w301) -> (refnum out=w296:refnum<file>, error out=w297:errorcluster)
            n198 = Close File(refnum=w296, error in=w297) -> ()  [unwired: 2 out]
          }
          frame #2 {
          }
        }
      }
      event "探头校正返回": Value Change {
        n199 = event-data() -> ()  [unwired: 1 in, 6 out]
        n200 = property on="窗格" class="Pane"("Origin"=T2 {"Horizontal"=0, "Vertical"=0} ("原点")) -> ()  [unwired: 2 in, 2 out]
        n201 = disable-structure shown="禁用" {
          disable-tunnel: w310 -> [w312 _]
          frame Disabled {
            n202 = for {
              tunnel: w312 -> [w315] mode=indexing
              n203 = property class="VI"(reference=w315) -> (reference out=w313:refnum<vi>, "Exec.State"=w314:T11)  [unwired: 1 in, 1 out]
              n204 = case shown="\"Run top level\"" w314 {
                tunnel: w313 -> [_ _ w316 w317]
                frame "Bad", Default {
                }
                frame "Idle" {
                }
                frame "Run top level" {
                  n205 = invoke class="VI" method="Abort VI"(reference=w316) -> ()  [unwired: 2 in, 3 out]
                }
                frame "Running" {
                  n206 = invoke class="VI" method="Abort VI"(reference=w317) -> ()  [unwired: 2 in, 3 out]
                }
              }
            }
          }
          frame Enabled {
          }
        }
      }
      event "探头校正": Value Change {
        n207 = event-data() -> ()  [unwired: 1 in, 6 out]
        n208 = property on="窗格" class="Pane"("Origin"=T2 {"Horizontal"=1656, "Vertical"=0} ("原点")) -> ()  [unwired: 2 in, 2 out]
        n209 = Index Array(array=w323, index=0 ("索引")) -> (element=w324:refnum<vi>)
        n210 = property class="VI"(reference=w324) -> (reference out=w319:refnum<vi>, "Exec.State"=w318:T11)  [unwired: 1 in, 1 out]
        n211 = case shown="\"Bad\", 默认" w318 {
          tunnel: [w326 w328] -> w322
          tunnel: w319 -> [w326 w327]
          frame "Bad", Default {
          }
          frame "Idle" {
            n212 = invoke class="VI" method="Run VI"(reference=w327, "Wait until done"=FALSE ("结束前等待"), "Auto Dispose Ref"=FALSE ("自动销毁引用")) -> (reference out=w328:refnum<vi>)  [unwired: 2 in, 4 out]
          }
        }
        n213 = invoke on="探头校准子面板" class="SubPnl" method="Remove VI"() -> (error out=w321:errorcluster)  [unwired: 3 in, 2 out]
        n214 = invoke on="探头校准子面板" class="SubPnl" method="Insert VI"(error in=w321, "VI Ref"=w322) -> ()  [unwired: 2 in, 4 out]
      }
      event "水温校准": Value Change {
        n215 = event-data() -> ()  [unwired: 1 in, 6 out]
        n216 = Index Array(array=w336, index=0 ("索引")) -> (element=w337:refnum<vi>)
        n217 = property class="VI"(reference=w337) -> (reference out=w332:refnum<vi>, "Exec.State"=w331:T11)  [unwired: 1 in, 1 out]
        n218 = case shown="\"Bad\", 默认" w331 {
          tunnel: [w338 w340] -> w334
          tunnel: w332 -> [w338 w339]
          frame "Bad", Default {
          }
          frame "Idle" {
            n219 = invoke class="VI" method="Run VI"(reference=w339, "Wait until done"=FALSE ("结束前等待"), "Auto Dispose Ref"=FALSE ("自动销毁引用")) -> (reference out=w340:refnum<vi>)  [unwired: 2 in, 4 out]
          }
        }
        n220 = invoke on="探头校准子面板" class="SubPnl" method="Remove VI"() -> (error out=w333:errorcluster)  [unwired: 3 in, 2 out]
        n221 = invoke on="探头校准子面板" class="SubPnl" method="Insert VI"(error in=w333, "VI Ref"=w334) -> ()  [unwired: 2 in, 4 out]
      }
      event "pH校准": Value Change {
        n222 = event-data() -> ()  [unwired: 1 in, 6 out]
        n223 = Index Array(array=w348, index=1 ("索引")) -> (element=w349:refnum<vi>)
        n224 = property class="VI"(reference=w349) -> (reference out=w344:refnum<vi>, "Exec.State"=w343:T11)  [unwired: 1 in, 1 out]
        n225 = case shown="\"Bad\", 默认" w343 {
          tunnel: w344 -> [w350 w354]
          tunnel: [w350 w351] -> w346
          frame "Bad", Default {
          }
          frame "Idle" {
            n226 = invoke class="VI" method="Run VI"(reference=w354, "Wait until done"=FALSE ("结束前等待"), "Auto Dispose Ref"=FALSE ("自动销毁引用")) -> (reference out=w351:refnum<vi>)  [unwired: 2 in, 4 out]
          }
        }
        n227 = invoke on="探头校准子面板" class="SubPnl" method="Remove VI"() -> (error out=w345:errorcluster)  [unwired: 3 in, 2 out]
        n228 = invoke on="探头校准子面板" class="SubPnl" method="Insert VI"(error in=w345, "VI Ref"=w346) -> ()  [unwired: 2 in, 4 out]
      }
      event "电导率校准": Value Change {
        n229 = event-data() -> ()  [unwired: 1 in, 6 out]
        n230 = Index Array(array=w360, index=2 ("索引")) -> (element=w361:refnum<vi>)
        n231 = property class="VI"(reference=w361) -> (reference out=w356:refnum<vi>, "Exec.State"=w355:T11)  [unwired: 1 in, 1 out]
        n232 = case shown="\"Bad\", 默认" w355 {
          tunnel: [w362 w364] -> w358
          tunnel: w356 -> [w362 w363]
          frame "Bad", Default {
          }
          frame "Idle" {
            n233 = invoke class="VI" method="Run VI"(reference=w363, "Wait until done"=FALSE ("结束前等待"), "Auto Dispose Ref"=FALSE ("自动销毁引用")) -> (reference out=w364:refnum<vi>)  [unwired: 2 in, 4 out]
          }
        }
        n234 = invoke on="探头校准子面板" class="SubPnl" method="Remove VI"() -> (error out=w357:errorcluster)  [unwired: 3 in, 2 out]
        n235 = invoke on="探头校准子面板" class="SubPnl" method="Insert VI"(error in=w357, "VI Ref"=w358) -> ()  [unwired: 2 in, 4 out]
      }
      event "溶解氧校准": Value Change {
        n236 = event-data() -> ()  [unwired: 1 in, 6 out]
        n237 = Index Array(array=w372, index=3 ("索引")) -> (element=w373:refnum<vi>)
        n238 = property class="VI"(reference=w373) -> (reference out=w368:refnum<vi>, "Exec.State"=w367:T11)  [unwired: 1 in, 1 out]
        n239 = case shown="\"Bad\", 默认" w367 {
          tunnel: [w374 w376] -> w370
          tunnel: w368 -> [w374 w375]
          frame "Bad", Default {
          }
          frame "Idle" {
            n240 = invoke class="VI" method="Run VI"(reference=w375, "Wait until done"=FALSE ("结束前等待"), "Auto Dispose Ref"=FALSE ("自动销毁引用")) -> (reference out=w376:refnum<vi>)  [unwired: 2 in, 4 out]
          }
        }
        n241 = invoke on="探头校准子面板" class="SubPnl" method="Remove VI"() -> (error out=w369:errorcluster)  [unwired: 3 in, 2 out]
        n242 = invoke on="探头校准子面板" class="SubPnl" method="Insert VI"(error in=w369, "VI Ref"=w370) -> ()  [unwired: 2 in, 4 out]
      }
      event "浊度校准": Value Change {
        n243 = event-data() -> ()  [unwired: 1 in, 6 out]
        n244 = Index Array(array=w384, index=4 ("索引")) -> (element=w385:refnum<vi>)
        n245 = property class="VI"(reference=w385) -> (reference out=w380:refnum<vi>, "Exec.State"=w379:T11)  [unwired: 1 in, 1 out]
        n246 = case shown="\"Bad\", 默认" w379 {
          tunnel: [w386 w388] -> w382
          tunnel: w380 -> [w386 w387]
          frame "Bad", Default {
          }
          frame "Idle" {
            n247 = invoke class="VI" method="Run VI"(reference=w387, "Wait until done"=FALSE ("结束前等待"), "Auto Dispose Ref"=FALSE ("自动销毁引用")) -> (reference out=w388:refnum<vi>)  [unwired: 2 in, 4 out]
          }
        }
        n248 = invoke on="探头校准子面板" class="SubPnl" method="Remove VI"() -> (error out=w381:errorcluster)  [unwired: 3 in, 2 out]
        n249 = invoke on="探头校准子面板" class="SubPnl" method="Insert VI"(error in=w381, "VI Ref"=w382) -> ()  [unwired: 2 in, 4 out]
      }
      event "叶绿素a校准": Value Change {
        n250 = event-data() -> ()  [unwired: 1 in, 6 out]
        n251 = Index Array(array=w396, index=5 ("索引")) -> (element=w397:refnum<vi>)
        n252 = property class="VI"(reference=w397) -> (reference out=w392:refnum<vi>, "Exec.State"=w391:T11)  [unwired: 1 in, 1 out]
        n253 = case shown="\"Bad\", 默认" w391 {
          tunnel: [w398 w400] -> w394
          tunnel: w392 -> [w398 w399]
          frame "Bad", Default {
          }
          frame "Idle" {
            n254 = invoke class="VI" method="Run VI"(reference=w399, "Wait until done"=FALSE ("结束前等待"), "Auto Dispose Ref"=FALSE ("自动销毁引用")) -> (reference out=w400:refnum<vi>)  [unwired: 2 in, 4 out]
          }
        }
        n255 = invoke on="探头校准子面板" class="SubPnl" method="Remove VI"() -> (error out=w393:errorcluster)  [unwired: 3 in, 2 out]
        n256 = invoke on="探头校准子面板" class="SubPnl" method="Insert VI"(error in=w393, "VI Ref"=w394) -> ()  [unwired: 2 in, 4 out]
      }
    }
  }
  n257 = while {
    tunnel: w9 -> [w404]
    stop <- FALSE stop-if-true
    n258 = Dequeue Element(queue=w404) -> (element=w403:string)  [unwired: 2 in, 3 out]
    n259 = case shown="\"close\"" w403 {
      tunnel: [_ w408 w413] -> _
      frame "假", Default {
      }
      frame "open" {
        n260 = global read "多参数全局变量.vi" "MB_Serial session"() -> (w407:refnum<class "MB_Master_Serial.lvclass">)
        n261 = global read "断电保存变量.vi" "VISA资源名称"() -> (w410:refnum<visa-resource-name>)
        n262 = call "close MB.vi"("MB_Serial session"=w407) -> ("error out"=w411:errorcluster)  [unwired: 10 in]
        n263 = call "open MB.vi"("error in (no error)"=w411, "Serial Config"=T15 {"baud rate (bps)"=9600, "stop bits"=10, "parity"=0, "flow control"=0, "timeout"=1000, "retries"=1}, "VISA资源名称"=w410) -> ("error out"=w408:errorcluster, "MB_Serial session"=w406:refnum<class "MB_Master_Serial.lvclass">)  [unwired: 7 in]
        n264 = global write "多参数全局变量.vi" "MB_Serial session"(w406) -> ()
      }
      frame "close" {
        n265 = global read "多参数全局变量.vi" "MB_Serial session"() -> (w412:refnum<class "MB_Master_Serial.lvclass">)
        n266 = call "close MB.vi"("MB_Serial session"=w412) -> ("error out"=w413:errorcluster)  [unwired: 10 in]
      }
    }
  }
